vi "Shutdown.vi"(8 "error in":errorcluster, 11 "Instrument in":refnum<class "Instrument.lvclass">) -> (0 "error out":errorcluster, 3 "Instrument out":refnum<class "Instrument.lvclass">)   [LabVIEW 2016, in "Instrument.lvclass"]
doc: "General Instrument shutdown procedures. Kill open queues."
uses:
  Instrument.lvclass
  Session APIs/Session Log/System Log.lvclass
  G:/sw_repo/For Builds/Reusable/Session APIs/_Session Fwk/Session - Root.lvclass
  Session APIs/File Access/Config Data/Config Data.lvclass
  Instrument.lvclass/Instrument.ctl
  Session APIs/_Session Fwk/Session - Root.lvclass
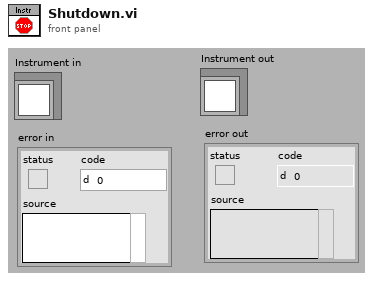
[diagram p1: front panel]
types:
  T1 = typedef "Session - Root.lvclass/Session Handle.ctl" = refnum<data-value>
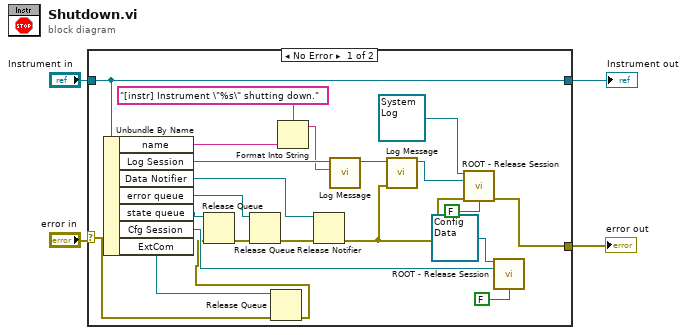
[diagram p0: block diagram]
diagram:
  n1 = case shown="No Error" "error in" {
    selector: "error in" -> [w6 w28]
    tunnel: [w22 w28] -> w3
    tunnel: [w26 w27] -> w1
    tunnel: "Instrument in" -> [w26 w27]
    frame No Error {
      n2 = Unbundle By Name(w26) -> ("name"=w16:string, "Log Session"=w19:T1, "Data Notifier"=w12:refnum<notifier>, "error queue"=w24:refnum<queue>, "state queue"=w25:refnum<queue>, "Cfg Session"=w9:T1, "ExtCom"=w7:refnum<queue>)
      n3 = Release Queue(queue=w7, error in (no error)=w6) -> (error out=w5:errorcluster)  [unwired: 1 in, 2 out]
      n4 = Release Queue(queue=w25, error in (no error)=w5) -> (error out=w23:errorcluster)  [unwired: 1 in, 2 out]
      n5 = Release Queue(queue=w24, error in (no error)=w23) -> (error out=w13:errorcluster)  [unwired: 1 in, 2 out]
      n6 = Format Into String(format string="[instr] Instrument \"%s\" shutting down.", w16) -> (resulting string=w14:string)  [unwired: 2 in, 1 out]
      n7 = Release Notifier(notifier=w12, error in (no error)=w13) -> (error out=w11:errorcluster)  [unwired: 1 in, 2 out]
      n8 = call "Log Message.vi"("MSG In"=w14, "session in"=w19) -> ("session out"=w18:T1)  [unwired: 8 in, 1 out]
      n9 = call "Log Message.vi"("error in"=w11, "session in"=w18) -> ("session out"=w17:T1)  [unwired: 8 in, 1 out]
      n10 = call "ROOT - Release Session.vi"("OBJ - Session in"=refnum<class "System Log.lvclass"> refnum ("Sys Log"), "Session Handle in"=w17, "error in (no error)"=w11, "force destroy? (F)"=FALSE) -> ("error out"=w22:errorcluster)  [unwired: 10 in, 1 out]
      n11 = call "ROOT - Release Session.vi"("OBJ - Session in"=refnum<class "Config Data.lvclass"> refnum ("Config Data"), "Session Handle in"=w9, "force destroy? (F)"=FALSE) -> ()  [unwired: 11 in, 2 out]
    }
    frame Error {
    }
  }
  "error out" <- w3
  "Instrument out" <- w1
